vi "Read Station Config.vi"(10 "Path to Config Folder":path, 11 "Application in":refnum<class "Application.lvclass">) -> (3 "Application out":refnum<class "Application.lvclass">)   [LabVIEW 2017, in "Application.lvlib" / "Application.lvclass"]
uses:
  Application.lvclass
  Station Config/Class/Station Config.lvclass
  Application.lvclass/Application.ctl
  Properties/App Properties.lvclass/App Properties.ctl
  Properties/App Properties.lvclass
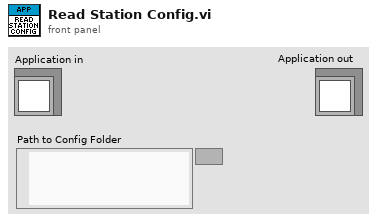
[diagram p1: front panel]
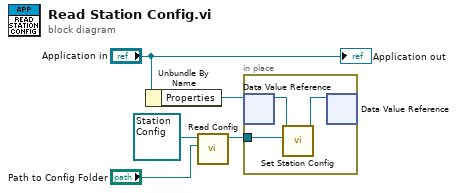
[diagram p0: block diagram]
diagram:
  n1 = Unbundle By Name("Application in") -> ("Properties"=w4:refnum<data-value>)
  n2 = call-dynamic "Read Config.vi"("Path to Config Folder"="Path to Config Folder", "Station Config in"=refnum<class "Station Config.lvclass"> refnum) -> ("Station Config out"=w5:refnum<class "Station Config.lvclass">)  [unwired: 8 in, 1 out]
  n3 = in-place {
    in-place-border: w5 -> [w6]
    n4 = in-place-dvr #1(w4) -> (w8:refnum<class "App Properties.lvclass">)  [unwired: 1 out]
    n5 = call "Set Station Config.vi"("Station Config"=w6, "App Properties in"=w8) -> ("App Properties out"=w7:refnum<class "App Properties.lvclass">)  [unwired: 8 in, 1 out]
    n6 = in-place-dvr #1(w7) -> ()  [unwired: 2 out]
  }
  "Application out" <- "Application in"
